vi "Solution.vi"() -> ()   [LabVIEW 2019]
uses:
  <vilib>/httpClient/POSTBuffer.vi
  <vilib>/httpClient/LabVIEWHTTPClient.lvlib
panel:
  out "error out":errorcluster
  out "Tab Control":enum32{"Page 1", "Page 2"}(tab)
  in  "API key":string="638j8h2379vbh32hjk56783jktrew761"
  in  "licenseHash":string="5d57e8bcc32f97663a8590781b39002d"
  in  "clientSerial":string="developer"
  in  "Authenticate":bool
  in  "Select Chip":string(combo)="001-190"
  in  "stop":bool
  out "ID":string
  out "Model":string
  out "Unit":string
  out "Label":string
  out "Value":string
  in  "Select Spec":string(combo)
  out "Created":dbl
  out "jwtToken":string="eyJhbGciOiJIUzI1NiIsInR5cCI6IkpXVCJ9.eyJkYXRhIjp7ImNsaWVudFNlcmlhbCI6ImRldmVsb3BlciIsImxpY2Vuc2VWYWxpZFVudGlsIjoiMTg5NzkxODUyNjAwMCJ9LCJpYXQiOjE1ODIzMDAyMjksImV4cCI6MTU4MjM4NjYyOX0.iY-YLVVzkOAtTILYIx_1T5l_p0eZNRgwxAISscrqsL8"
  # "Authentication"
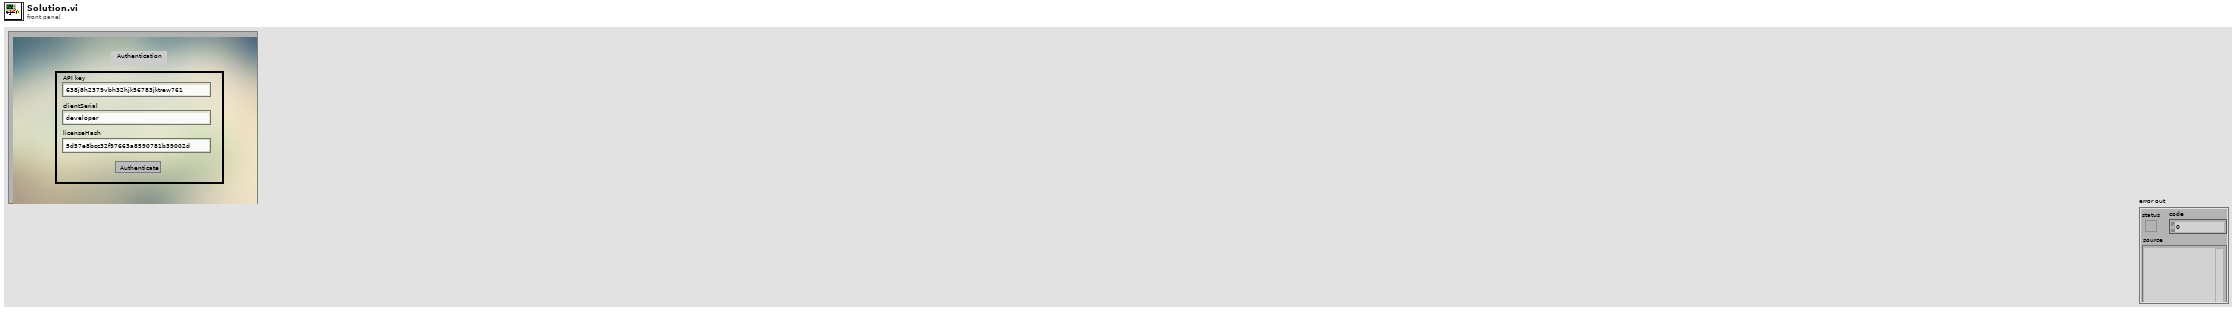
[diagram p1: front panel]
types:
  T1 = cluster{"clientSerial":string, "licenseHash":string}
  T2 = typedef "LabVIEWHTTPClient.lvlib/ClientHandle.ctl" = refnum<k1>
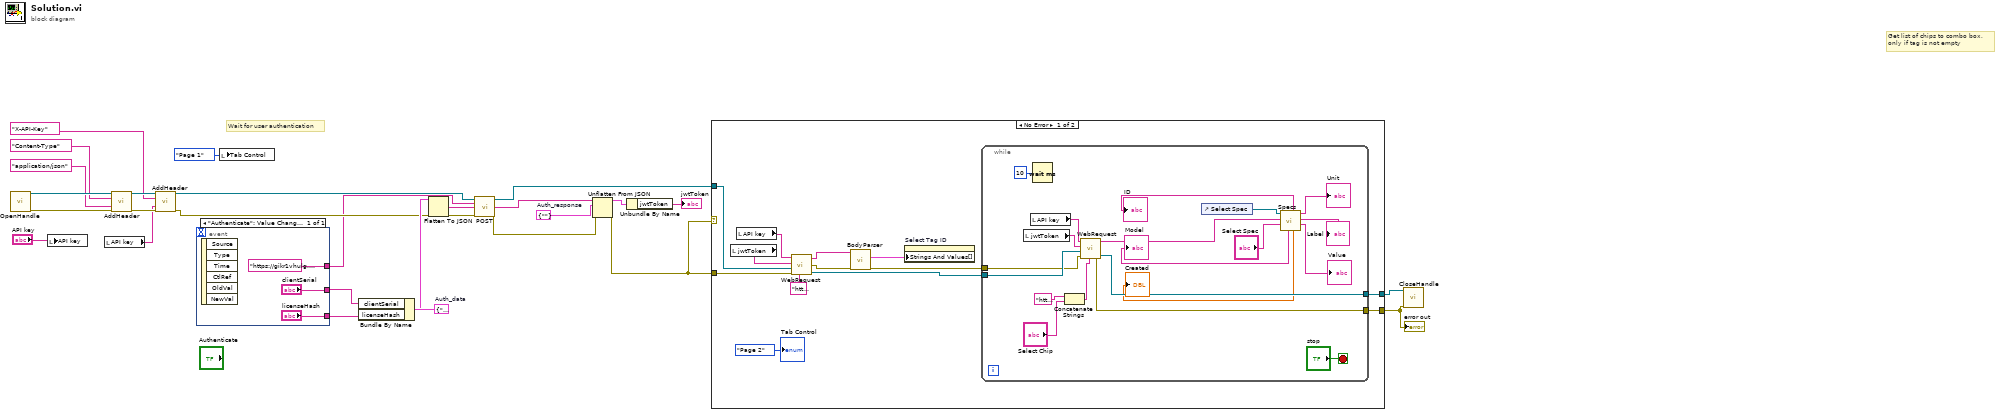
[diagram p0: block diagram]
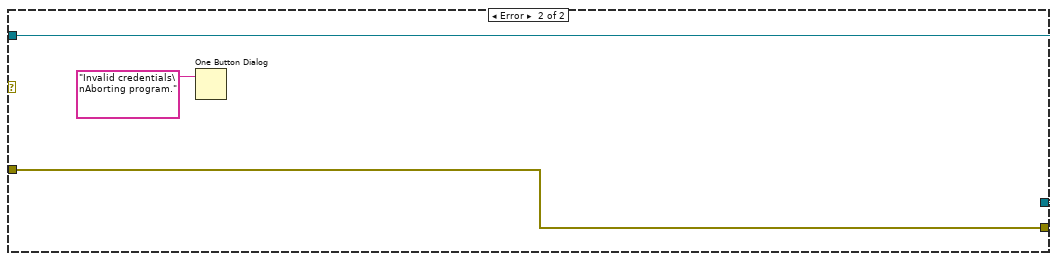
[diagram p2: hidden frame]
diagram:
  w18 = cluster{"jwtToken":string} {"jwtToken"=""}  # Auth_response
  w21 = T1 {"clientSerial"="", "licenseHash"=""}  # Auth_data
  # "Wait for user authentication"
  # "Get list of chips to combo box,\nonly if tag is not empty"
  n1 = call <vilib>:"OpenHandle.vi"() -> ("client handle out"=w28:T2, "error out"=w27:errorcluster)  [unwired: 14 in]
  n2 = local write "API key"("API key") -> ()
  n3 = local read "API key"() -> (w11:string)
  n4 = call <vilib>:"AddHeader.vi"("client handle"=w28, "header"="Content-Type", "value"="application/json", "error in (no error)"=w27) -> ("client handle out"=w24:T2, "error out"=w23:errorcluster)  [unwired: 10 in]
  n5 = call <vilib>:"AddHeader.vi"("client handle"=w24, "header"="X-API-Key", "value"=w11, "error in (no error)"=w23) -> ("client handle out"=w7:T2, "error out"=w8:errorcluster)  [unwired: 10 in]
  n6 = event shown="[0] \"Authenticate\": Value Change" {
    selector: _ -> [_]
    dyn-events: _ -> [_]
    timeout: _ -> [_]
    tunnel: ["https://gikr1vhulg.execute-api.eu-west-1.amazonaws.com/playground/v1/auth/client"] -> w5
    tunnel: ["clientSerial"] -> w4
    tunnel: ["licenseHash"] -> w3
    event "Authenticate": Value Change {
      n7 = event-data() -> ()  [unwired: 1 in, 6 out]
    }
  }
  n8 = local write "Tab Control"(enum32{"Page 1", "Page 2"}."Page 1" ("Tab Control")) -> ()
  n9 = Bundle By Name(cluster=w21, "clientSerial"=w4, "licenseHash"=w3) -> (w14:T1)
  n10 = Flatten To JSON(anything=w14, error in (no error)=w8) -> (JSON string=w20:string, 11:w15:errorcluster)  [unwired: 1 in]
  n11 = call-poly <vilib>:"POST.vi"("client handle"=w7, "url"=w5, "buffer"=w20, "error in (no error)"=w15) -> ("client handle out"=w13:T2, "body"=w19:string, "error out"=w10:errorcluster)  [unwired: 8 in, 1 out]
  n12 = Unflatten From JSON(JSON string=w19, type and defaults=w18, error in (no error)=w10) -> (value=w17:cluster{"jwtToken":string}, error out=w9:errorcluster)  [unwired: 4 in]
  n13 = Unbundle By Name(w17) -> ("jwtToken"=→"jwtToken":string)
  n14 = case shown="No Error" w9 {
    tunnel: w13 -> [w41 w66]
    tunnel: w9 -> [w40 w65]
    tunnel: [w33 w66] -> w2
    tunnel: [w32 w65] -> w1
    frame No Error {
      n15 = local read "jwtToken"() -> (w42:string)
      n16 = local read "API key"() -> (w43:string)
      n17 = call "WebRequest.vi"("API Key"=w43, "JWT Token"=w42, "client handle in"=w41, "URL"="https://gikr1vhulg.execute-api.eu-west-1.amazonaws.com/playground/v1/chips/tags", "error in (no error)"=w40) -> ("body"=w37:string, "error out"=w38:errorcluster, "client handle out"=w36:T2)  [unwired: 1 in]
      n18 = call "BodyParser.vi"("error in (no error)"=w38, "body"=w37) -> ("error out"=w35:errorcluster, "Array"=w44:cluster{"id":string, string}[])  [unwired: 7 in, 1 out]
      n19 = property on="Select Tag ID" class="CmbBox"("Strings And Values[]"=w44) -> ()  [unwired: 2 in, 2 out]
      n20 = while {
        tunnel: w36 -> [w57]
        tunnel: [w58] -> w33
        tunnel: [w55] -> w32
        tunnel: w35 -> [w56]
        stop <- "stop" stop-if-true
        n21 = local read "jwtToken"() -> (w63:string)
        n22 = local read "API key"() -> (w62:string)
        n23 = Wait (ms)(milliseconds to wait=u32 10) -> ()  [unwired: 1 out]
        n24 = Concatenate Strings("https://gikr1vhulg.execute-api.eu-west-1.amazonaws.com/playground/v1/chips/tags/", "Select Chip") -> (w59:string)
        n25 = call "WebRequest.vi"("API Key"=w62, "JWT Token"=w63, "client handle in"=w57, "URL"=w59, "error in (no error)"=w56) -> ("body"=w54:string, "error out"=w55:errorcluster, "client handle out"=w58:T2)  [unwired: 1 in]
        n26 = control-ref of="Select Spec"() -> (w51:refnum<vi>)
        n27 = call "Specs.vi"("Select Spec"="Select Spec", "body"=w54, "ComboBox in"=w51) -> ("Value"=→"Value":string, "Label"=→"Label":string, "Unit"=→"Unit":string, "Created"=→"Created":dbl, "ID"=→"ID":string, "Model"=→"Model":string)  [unwired: 3 in]
      }
      "Tab Control" <- enum32{"Page 1", "Page 2"}."Page 2" ("Tab Control")
    }
    frame Error {
      n28 = One Button Dialog(message="Invalid credentials\nAborting program.") -> ()  [unwired: 1 in, 1 out]
    }
  }
  "error out" <- w1
  n29 = call <vilib>:"CloseHandle.vi"("client handle"=w2, "error in (no error)"=w1) -> ()  [unwired: 13 in, 1 out]
